vi "Get Variant Message.vi"(8 "error in (no error)":errorcluster, 11 "Message String in":refnum<class "Message String.lvclass">) -> (0 "error out":errorcluster, 1 "Value":variant, 2 "Name":string, 3 "Message String out":refnum<class "Message String.lvclass">)   [LabVIEW 2016, in "Stream Mediator.lvlib" / "Message String.lvclass"]
doc: "--\nCopyright © 2017 Composed SystemsI All rights reserved.\n\nAuthor: Jon McBee <jon.mcbee@composed.io>\n\nThis library is provided \"AS IS\" ,WITHOUT WARRANTIES OR\nCONDITIONS OF ANY KIND, either express or implied.\n\nComposed Systems -- composed.io\n\nStream 0.0.1.1\nJon McBee - Composed Systems\nCopyright (c) 2017, Composed Systems"
uses:
  <userlib>/Composed Systems/Stream/Mediator/Classes/Message String/Message String.lvclass
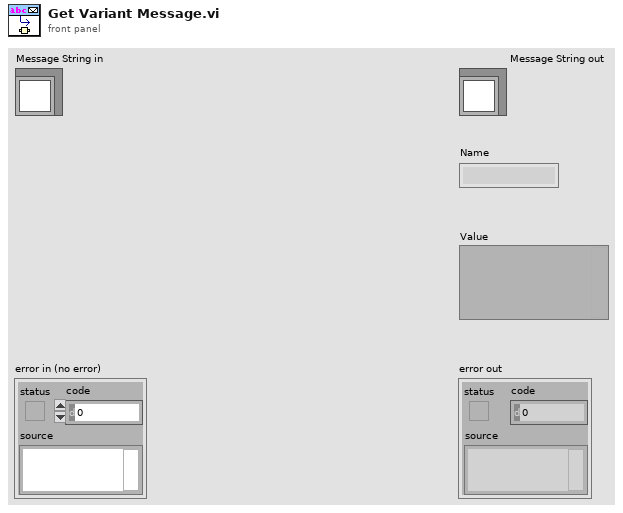
[diagram p1: front panel]
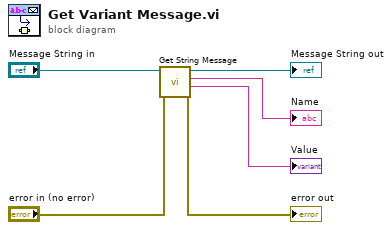
[diagram p0: block diagram]
diagram:
  n1 = call <userlib>:"Get String Message.vi"("error in (no error)"="error in (no error)", "Message String in"="Message String in") -> ("error out"=→"error out":errorcluster, "Value"=→"Value":string, "Name"=→"Name":string, "Message String out"=→"Message String out":refnum<class "Message String.lvclass">)  [unwired: 6 in]
